vi "Mathcad Close.vi"(8 "Error In":errorcluster, 10 "Exit Mathcad?":bool, 11 "Mathcad Reference":T1) -> (0 "Error Out":errorcluster)   [LabVIEW 2015]
doc: "Closes a Mathcad Reference that was opened by Mathcad Opens.vi. This will close the current open Mathcad Worksheet and (if \"Exit Mathcad?\" is set to True) will close the Mathcad Application as well.\n\nInputs\nMathcad Reference (Cluster- 3 Elements)\n Application Reference - Reference to the opened (parent) Mathcad Appliction Environement\n Worsheets Reference- Reference to the Worsheets Reference which is parent to the Worksheet Reference.\n Worksheet Reference- Reference to the Mathcad Worksheet Reference opened by the Mathcad_File_Open.vi\n \nExit Mathcad?-If True, closes the Mathcad Application Reference that was opened by Mathcad Open.vi. If you set this to False, you can re-retrieve the opened Mathcad Application Reference by calling Mathcad Open, again.\n\nError In- Error Cluster\n\nOutputs\n(only error out)"
uses:
  Mathcad Reference.ctl
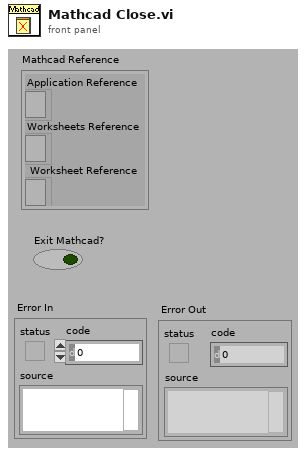
[diagram p1: front panel]
types:
  T1 = typedef "Mathcad Reference.ctl" = cluster{"Application Reference":refnum<k7>, "Worksheets Reference":refnum<k7>, " Worksheet Reference":refnum<k7>}
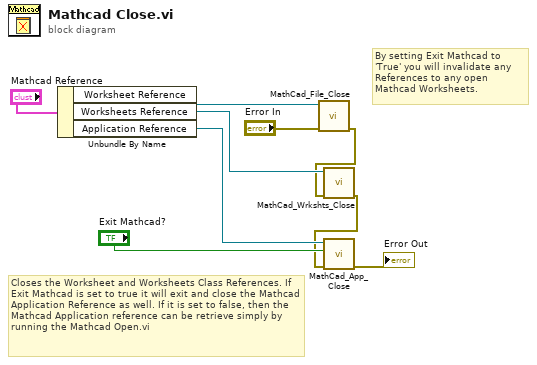
[diagram p0: block diagram]
diagram:
  # "By setting Exit Mathcad to 'True' you will invalidate any References to any open Mathcad Worksheets."
  # "Closes the Worksheet and Worksheets Class References. If Exit Mathcad is set to true it will exit and close the Mathcad Application Reference as well. If it is set to false, then the Mathcad Application reference can be retrieve simply by running the Mathcad Open.vi"
  n1 = Unbundle By Name("Mathcad Reference") -> ("Worksheet Reference"=w6:refnum<k7>, "Worksheets Reference"=w8:refnum<k7>, "Application Reference"=w7:refnum<k7>)
  n2 = call "MathCad_File_Close.vi"("error in (no error)"="Error In", "Mathcad Worksheet"=w6) -> ("error out"=w4:errorcluster)  [unwired: 9 in]
  n3 = call "MathCad_Wrkshts_Close.vi"("error in"=w4, "Worksheets Reference"=w8) -> ("error out"=w3:errorcluster)  [unwired: 9 in]
  n4 = call "MathCad_App_Close.vi"("error in (no error)"=w3, "Hide Only (don't Close)"="Exit Mathcad?", "Mathcad Application Reference"=w7) -> ("error out (no error)"=→"Error Out":errorcluster)  [unwired: 8 in]
